vi "read from file.vi"(5 "File Path":path) -> (0 "Delay Info":T1, 1 "Spectrum Info":T2, 2 "Experiment Trace":dbl[][](array[numeric]))   [LabVIEW 2013]
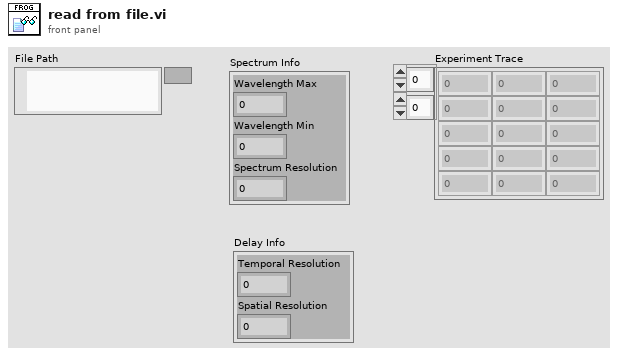
[diagram p1: front panel]
types:
  T1 = cluster{"Temporal Resolution":u16, "Spatial Resolution":u16}
  T2 = cluster{"Wavelength Max":dbl, "Wavelength Min":dbl, "Spectrum Resolution":u16}
  T3 = cluster{"Temporal Resolution":u16, "Spatial Resolution (nm)":u16}
  T4 = cluster{"Wavelength Max (nm)":dbl, "Wavelength Min (nm)":dbl, "Spectrum Resolution":u16}
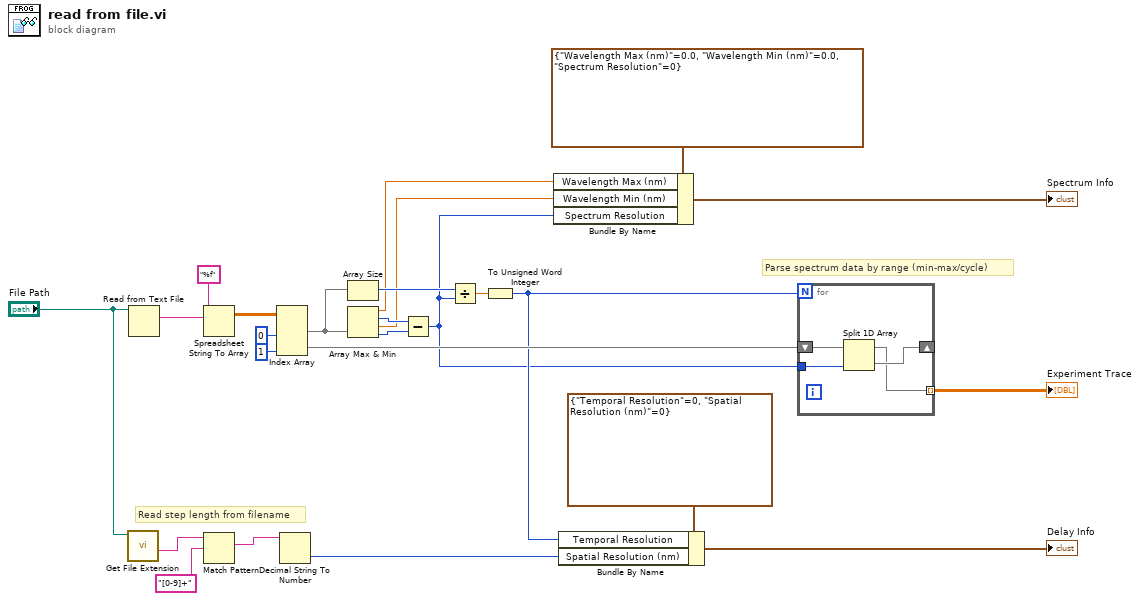
[diagram p0: block diagram]
diagram:
  # "Read step length from filename"
  # "Parse spectrum data by range (min-max/cycle)"
  n1 = call <vilib>:"Get File Extension.vi"("file"="File Path") -> ("filename without extension"=w12:string)  [unwired: 7 in, 3 out]
  n2 = Read from Text File(file (use dialog)="File Path") -> (text=w16:string)  [unwired: 3 in, 3 out]
  n3 = Spreadsheet String To Array(format string="%f", spreadsheet string=w16) -> (array=w18:dbl[][])  [unwired: 2 in]
  n4 = Match Pattern(string=w12, regular expression="[0-9]+") -> (match substring=w10:string)  [unwired: 1 in, 3 out]
  n5 = Index Array(array=w18, index (col) #1=0 ("disabled index (col)"), index (col) #2=1 ("index (col)")) -> (element #1=w21:dbl[], element #2=w22:dbl[])  [unwired: 2 in]
  n6 = Decimal String To Number(string=w10) -> (number=w2:i32)  [unwired: 2 in, 1 out]
  n7 = Array Size(array=w21) -> (size(s)=w25:i32)
  n8 = Array Max & Min(array=w21) -> (max value=w5:dbl, max index (indices)=w23:i32, min value=w4:dbl, min index (indices)=w24:i32)
  n9 = Subtract(x=w23, y=w24) -> (x-y=w6:i32)
  n10 = Divide(x=w25, y=w6) -> (x/y=w15:dbl)
  n11 = To Unsigned Word Integer(number=w15) -> (unsigned 16bit integer=w7:u16)
  n12 = Bundle By Name(cluster=T4 {"Wavelength Max (nm)"=0.0, "Wavelength Min (nm)"=0.0, "Spectrum Resolution"=0}, "Wavelength Max (nm)"=w5, "Wavelength Min (nm)"=w4, "Spectrum Resolution"=w6) -> (→"Spectrum Info":T4)
  n13 = Bundle By Name(cluster=T3 {"Temporal Resolution"=0, "Spatial Resolution (nm)"=0}, "Temporal Resolution"=w7, "Spatial Resolution (nm)"=w2) -> (→"Delay Info":T3)
  n14 = for {
    N: w7 -> [_]
    shift-right: [w28] -> _
    shift-left: w22 -> [w29]
    tunnel: [w27] -> w1 mode=indexing
    tunnel: w6 -> [w26]
    n15 = Split 1D Array(array=w29, index=w26) -> (first subarray=w27:dbl[], second subarray=w28:dbl[])
  }
  "Experiment Trace" <- w1
